vi "SubConfocal_StartStop.vi"(7 "Confocal scanner":T1={"SDC shutter"=FALSE, "Filter wheel"=3, "FW speed"=3, "Disk spinning"=FALSE, "Disk speed (rpm)"=3000.0} {"Disk speed (rpm)" min=1500.0 max=10000.0; "FW speed" min=1 max=5 step=1; "Filter wheel" items=["CFP"=1, "GFP"=2, "mCherry"=3, "Alexa-647"=4, "OFP"=5, "empty"=6]}, 8 "Error In":errorcluster, 11 "Confocal line (VISA IN)":refnum<visa-resource-name>="COM1") -> (0 "Error out":errorcluster)   [LabVIEW 2015]
panel:
  # "If no confocal scanner input, then stop by default."
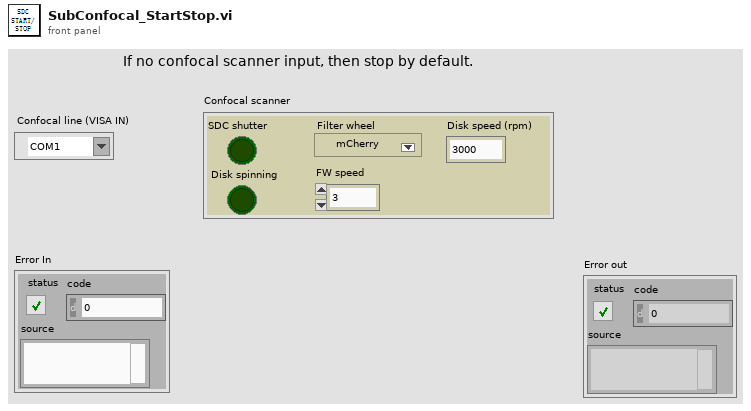
[diagram p1: front panel]
types:
  T1 = cluster{"SDC shutter":bool, "Filter wheel":u16, "FW speed":i32, "Disk spinning":bool, "Disk speed (rpm)":dbl}
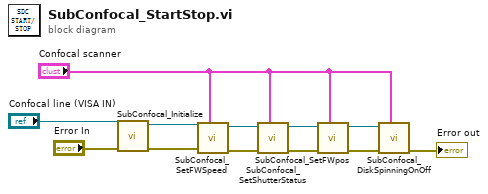
[diagram p0: block diagram]
diagram:
  n1 = call "SubConfocal_Initialize.vi"("error in"="Error In", "VISA  IN"="Confocal line (VISA IN)") -> ("error out"=w6:errorcluster, "VISA OUT"=w5:refnum<visa-resource-name>)  [unwired: 8 in]
  n2 = call "SubConfocal_SetFWSpeed.vi"("Confocal scanner"="Confocal scanner", "Error In"=w6, "Confocal line  (VISA IN)"=w5) -> ("Error out"=w7:errorcluster, "VISA OUT"=w8:refnum<visa-resource-name>)  [unwired: 7 in]
  n3 = call "SubConfocal_SetShutterStatus.vi"("Confocal scanner"="Confocal scanner", "Error In"=w7, "Confocal line (VISA IN)"=w8) -> ("Error out"=w12:errorcluster, "VISA OUT"=w11:refnum<visa-resource-name>)  [unwired: 7 in]
  n4 = call "SubConfocal_SetFWpos.vi"("Confocal scanner"="Confocal scanner", "Error In"=w12, "Confocal line (VISA IN)"=w11) -> ("Error out"=w10:errorcluster, "VISA OUT"=w9:refnum<visa-resource-name>)  [unwired: 7 in]
  n5 = call "SubConfocal_DiskSpinningOnOff.vi"("Confocal scanner"="Confocal scanner", "Error In"=w10, "Confocal line (VISA IN)"=w9) -> ("Error out"=→"Error out":errorcluster)  [unwired: 7 in, 1 out]
